vi "COB Receive.vi"(8 "error in":errorcluster, 11 "CAN Task in":refnum<class "CANopen Task Actor.lvclass">) -> (0 "error out":errorcluster, 1 "Data":u8[](array[numeric]) format="%.0x", 2 "CAN-ID":u32 format="%.0x", 3 "CAN Task out":refnum<class "CANopen Task Actor.lvclass">, 4 "No Data?":bool)   [LabVIEW 2024, in "CANopen Task Actor.lvlib" / "CANopen Task Actor.lvclass"]
uses:
  CANopen Task Actor.lvclass
  CANopen Task Actor.lvclass/CANopen Task Actor.ctl
  HAL/HAL/Protocols/ICAN/ICAN.lvclass
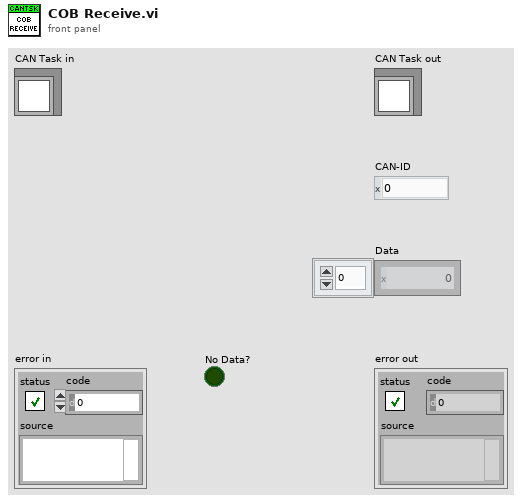
[diagram p1: front panel]
types:
  T1 = cluster{"ID":u32, "MSG type":u8, "DLC":u8, "Time Stamp":timestamp, "DATA":u8[]}
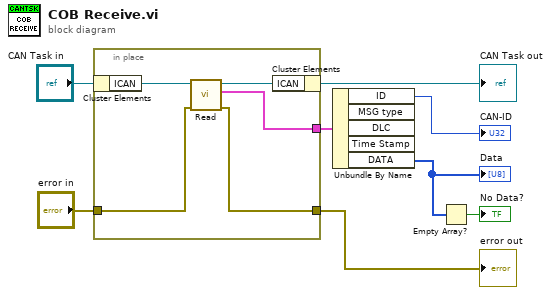
[diagram p0: block diagram]
diagram:
  n1 = in-place {
    in-place-border: "error in" -> [w10]
    in-place-border: [w11] -> w6
    in-place-border: [w9] -> w5
    n2 = in-place-cluster #1("CAN Task in") -> ("ICAN"=w13:refnum<class "ICAN.lvclass">)
    n3 = call-dynamic "Read.vi"("error in (no error)"=w10, "ICAN in"=w13) -> ("error out"=w11:errorcluster, "CAN Message"=w9:T1, "ICAN out"=w12:refnum<class "ICAN.lvclass">)  [unwired: 7 in]
    n4 = in-place-cluster #1("ICAN"=w12) -> (→"CAN Task out":refnum<class "CANopen Task Actor.lvclass">)
  }
  "error out" <- w6
  n5 = Unbundle By Name(w5) -> ("ID"=→"CAN-ID":u32, "DATA"=w1:u8[])  [unwired: 3 out]
  "Data" <- w1
  n6 = Empty Array?(array=w1) -> (empty?=→"No Data?":bool)
